vi "TCP Write Stream.vi"(5 "file dialog info":T1={"prompt"="Please select a file to read from", "pattern"="*", "default name"="", "start path"=path ""}, 6 "chunk size (32768)":i64=32768, 7 "binary":bool=TRUE, 8 "error in (no error)":errorcluster, 9 "data":string, 10 "data file (<NAP>)":path=path "", 11 "connection":refnum<k5>) -> (0 "error out":errorcluster, 1 "bytes written":i64, 2 "data file out":path, 3 "duplicate connection":refnum<k5>, 4 "file error":errorcluster)   [LabVIEW 2020, in "NI_FTP.lvlib"]
doc: "Write all data to a TCP.\nIf \"data file\" is specified, its contents are written, otherwise \"data\" is used.\nIf \"binary\" is FALSE, EOLN characters in the data will be replaced with CRLF..\n\"chunk size\" determines how many bytes at a time are read from the file"
uses:
  <vilib>/FTP/NI_FTP.lvlib
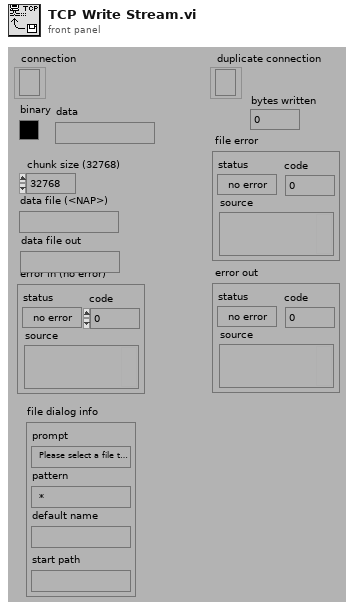
[diagram p1: front panel]
types:
  T1 = cluster{"prompt":string, "pattern":string, "default name":string, "start path":path}
  T2 = enum16{"read/write", "read-only", "write-only", "write-only (truncate)"}
  T3 = enum16{"open", "open or create", "create or replace", "create"}
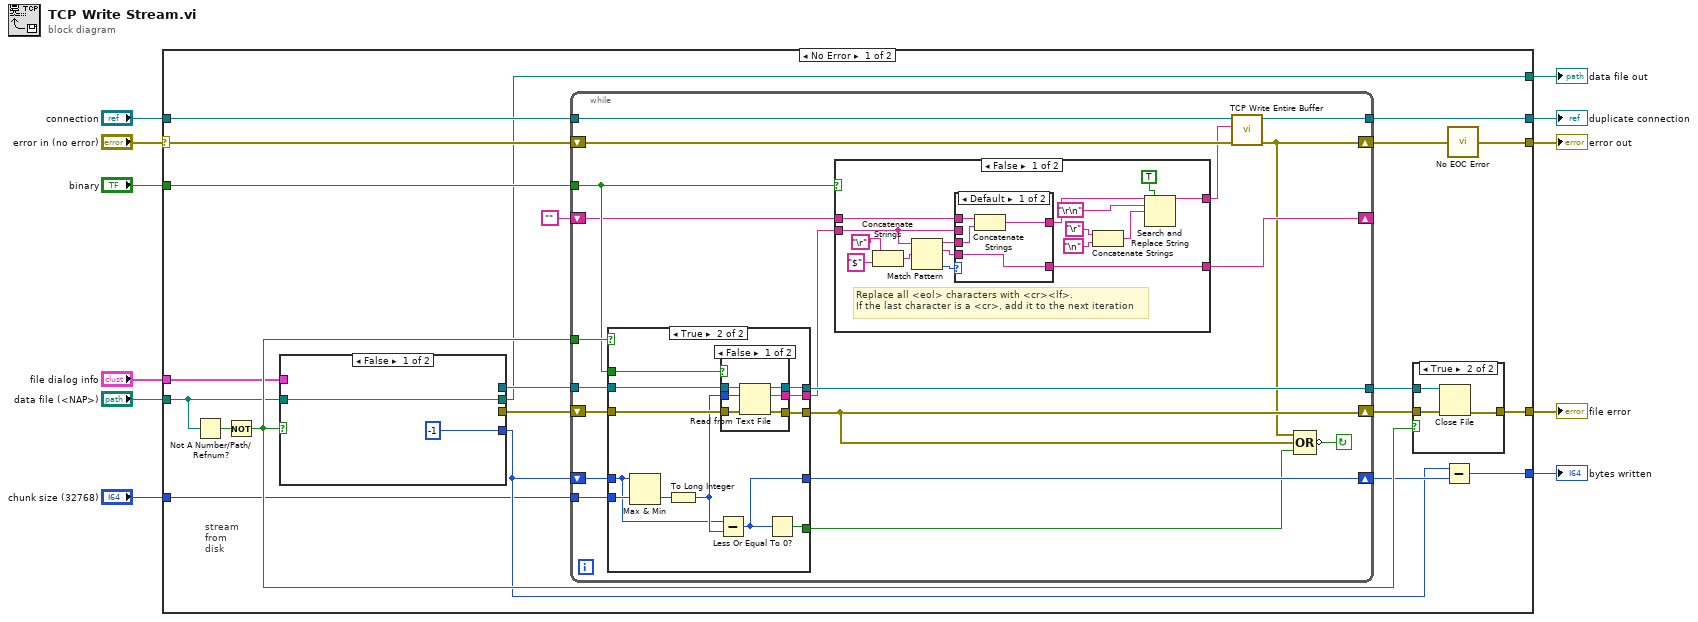
[diagram p0: block diagram]
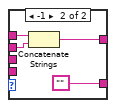
[diagram p2: hidden frame]
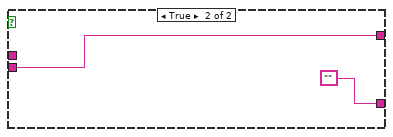
[diagram p3: hidden frame]
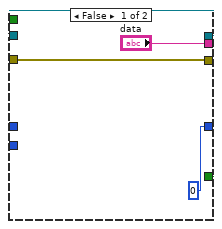
[diagram p4: hidden frame]
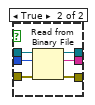
[diagram p5: hidden frame]
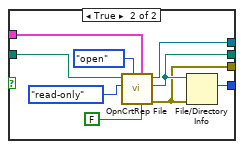
[diagram p7: hidden frame]
diagram:
  n1 = case shown="No Error" "error in (no error)" {
    selector: "error in (no error)" -> [w17 w122]
    tunnel: [w28 w122] -> w11
    tunnel: [w27 w123] -> w10
    tunnel: [w23 _] -> w9
    tunnel: [w19 _] -> w8
    tunnel: "connection" -> [w18 w123]
    tunnel: "data file (<NAP>)" -> [w16 _]
    tunnel: "chunk size (32768)" -> [w15 _]
    tunnel: "file dialog info" -> [w14 _]
    tunnel: "binary" -> [w13 _]
    tunnel: [w12 _] -> w1
    frame No Error {
      # "stream from disk"
      n2 = Not A Number/Path/Refnum?(number/path/refnum=w16) -> (NaN/Path/Refnum?=w30:bool)
      n3 = Not(x=w30) -> (.not. x?=w26:bool)
      n4 = case shown="False" w26 {
        tunnel: w16 -> [w111 w121]
        tunnel: [_ w118] -> w32
        tunnel: [_ w117] -> w31
        tunnel: [i64 -1 ("size") w114] -> w20
        tunnel: [w111 w119] -> w12
        tunnel: w14 -> [_ w113]
        frame False {
        }
        frame True {
          n5 = call <vilib>:"OpnCrtRep File.vi"("advisory dialog? (display:T)"=FALSE, "file dialog info"=w113, "function (open:0)"=T3."open", "open mode (0)"=T2."read-only", "file path"=w121) -> ("error out"=w117:errorcluster, "new file path"=w119:path, "refnum"=w118:refnum<file>)  [unwired: 3 in, 1 out]
          n6 = File/Directory Info(path=w119, error in=w117) -> (size=w114:i64)  [unwired: 6 out]
        }
      }
      n7 = while {
        shift-left: w20 -> [w43]
        shift-right: [w42] -> w22
        tunnel: [w44] -> w24
        tunnel: [w46] -> w27
        tunnel: w18 -> [w47]
        tunnel: w13 -> [w41]
        tunnel: w26 -> [w50]
        shift-left: w17 -> [w51]
        shift-right: [w34] -> w29
        shift-left: w31 -> [w49]
        shift-right: [w35] -> w25
        tunnel: w32 -> [w48]
        shift-right: [w38] -> _
        shift-left: "" -> [w39]
        tunnel: w15 -> [w36]
        stop <- w45 continue-if-true
        n8 = case shown="True" w50 {
          tunnel: w49 -> [w82 w93]
          tunnel: [w82 w89] -> w35
          tunnel: w41 -> [_ w94]
          tunnel: w48 -> [w81 w92]
          tunnel: [w81 w90] -> w44
          tunnel: ["data" w91] -> w40
          tunnel: [TRUE w87] -> w33
          tunnel: w43 -> [_ w83]
          tunnel: [i64 0 w88] -> w42
          tunnel: w36 -> [_ w84]
          frame False {
          }
          frame True {
            n9 = Max & Min(x=w83, y=w84) -> (min(x,y)=w86:i64)  [unwired: 1 out]
            n10 = To Long Integer(number=w86) -> (32bit integer=w85:i32)
            n11 = Subtract(x=w83, y=w85) -> (x-y=w88:i64)
            n12 = case shown="False" w94 {
              tunnel: [w99 w106] -> w89
              tunnel: w93 -> [w100 w105]
              tunnel: w85 -> [w96 w104]
              tunnel: w92 -> [w97 w103]
              tunnel: [w98 w102] -> w90
              tunnel: [w95 w101] -> w91
              frame False {
                n13 = Read from Text File(file (use dialog)=w97, count=w96, error in=w100) -> (refnum out=w98:refnum<file>, text=w95:string, error out=w99:errorcluster)  [unwired: 2 out]
              }
              frame True {
                n14 = Read from Binary File(8:w105, 10:w104, 11:w103) -> (0:w106:errorcluster, 2:w101:string, 3:w102:refnum<file>)  [unwired: 4 out]
              }
            }
            n15 = Less Or Equal To 0?(x=w88) -> (x <= 0?=w87:bool)
          }
        }
        n16 = case shown="False" w41 {
          tunnel: w40 -> [w64 w76]
          tunnel: w39 -> [w63 _]
          tunnel: [w62 ""] -> w38
          tunnel: [w55 w76] -> w37
          frame False {
            # "Replace all <eol> characters with <cr><lf>.\nIf the last character is a <cr>, add it to the next iteration"
            n17 = Concatenate Strings("\r", "$" ("string")) -> (w54:string)
            n18 = Match Pattern(string=w64, regular expression=w54) -> (before substring=w66:string, match substring=w67:string, offset past match=w65:i32)  [unwired: 2 out]
            n19 = case shown="Default" w65 {
              tunnel: w63 -> [w71 w74]
              tunnel: [w68 ""] -> w62
              tunnel: w64 -> [_ w73]
              tunnel: [w69 w72] -> w61
              tunnel: w66 -> [w70 _]
              tunnel: w67 -> [w68 _]
              frame Default {
                n20 = Concatenate Strings(w71, w70) -> (w69:string)
              }
              frame -1 {
                n21 = Concatenate Strings(w74, w73) -> (w72:string)
              }
            }
            n22 = Concatenate Strings("\r", "\n") -> (w56:string)
            n23 = Search and Replace String(replace all?=TRUE ("replace all? (F)"), input string=w61, search string="\r\n", replace string=w56) -> (result string=w55:string)  [unwired: 1 in, 6 out]
          }
          frame True {
          }
        }
        n24 = call <vilib>:"TCP Write Entire Buffer.vi"("error in (no error)"=w51, "data in"=w37, "connection ID"=w47) -> ("error out"=w34:errorcluster, "connection ID out"=w46:refnum<k5>)  [unwired: 7 out]
        n25 = Compound Arithmetic op=OR(w34, w35, w33) -> (invert w45:bool)
      }
      n26 = case shown="True" w26 {
        tunnel: w25 -> [w107 w110]
        tunnel: w24 -> [_ w109]
        tunnel: [w107 w108] -> w23
        frame False {
        }
        frame True {
          n27 = Close File(refnum=w109, error in=w110) -> (error out=w108:errorcluster)  [unwired: 1 out]
        }
      }
      n28 = Subtract(x=w20, y=w22) -> (x-y=w19:i64)
      n29 = call <vilib>:"No EOC Error.vi"("error in (no error)"=w29) -> ("error out"=w28:errorcluster)  [unwired: 4 out]
    }
    frame Error {
    }
  }
  "error out" <- w11
  "duplicate connection" <- w10
  "file error" <- w9
  "bytes written" <- w8
  "data file out" <- w1
